vi "SUB_OUT_SpaceString_token.vi"(3 "input string":string) -> (1 "result string":string)   [LabVIEW 2011]
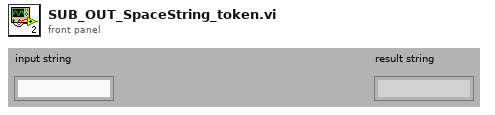
[diagram p1: front panel]
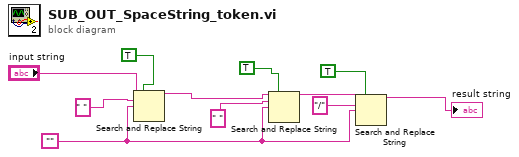
[diagram p0: block diagram]
diagram:
  w3 = ""
  n1 = Search and Replace String(replace all?=TRUE ("replace all? (F)"), input string="input string", search string=" ", replace string=w3) -> (result string=w11:string)  [unwired: 4 in, 3 out]
  n2 = Search and Replace String(replace all?=TRUE ("ignore case? (F)"), input string=w11, search string=" ", replace string=w3) -> (result string=w5:string)  [unwired: 4 in, 3 out]
  n3 = Search and Replace String(replace all?=TRUE ("replace all? (F)"), input string=w5, search string="/", replace string=w3) -> (result string=→"result string":string)  [unwired: 4 in, 3 out]
